vi "multiple_food.vi"(11 "pieceOfWorld in":T2[][](array[typedef])) -> (1 "columns":i32[](array[numeric]), 2 "rows":i32[](array[numeric]), 3 "foodAmount":T1)   [LabVIEW 2015, in "PolyVIEW.lvclass"]
uses:
  PolyVIEW.lvclass
  actors/world/typedefs/worldCell_cluster.ctl
  actors/world/typedefs/markValue_cluster.ctl
  actors/world/typedefs/markValue.ctl
  actors/world/typedefs/markVolume.ctl
  actors/world/typedefs/amountOfFood.ctl
  actors/world/typedefs/anthillType_enum.ctl
  actors/world/world.lvlib
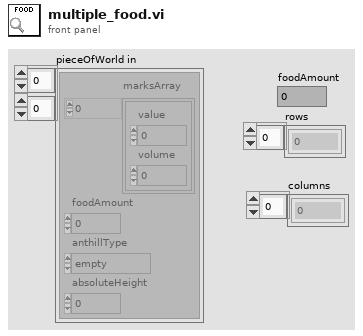
[diagram p1: front panel]
types:
  T1 = typedef "world.lvlib/amountOfFood.ctl" = i32
  T2 = typedef "world.lvlib/worldCell_cluster.ctl" = cluster{"marksArray":T3[], "foodAmount":T1, "anthillType":T6, "absoluteHeight":u8}
  T3 = typedef "world.lvlib/markValue_cluster.ctl" = cluster{"value":T4, "volume":T5}
  T4 = typedef "world.lvlib/markValue.ctl" = u8
  T5 = typedef "world.lvlib/markVolume.ctl" = u16
  T6 = typedef "world.lvlib/anthillType_enum.ctl" = enum16{"empty", "own", "rival"}
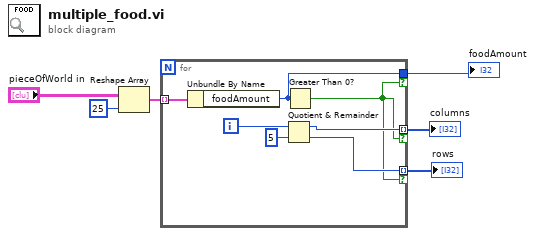
[diagram p0: block diagram]
diagram:
  n1 = Reshape Array("pieceOfWorld in", 25 ("dimension size")) -> (w5:T2[])
  n2 = for {
    tunnel: w5 -> [w13] mode=indexing
    tunnel: [w12] -> w3 if=w7
    tunnel: [w9] -> w2 mode=indexing if=w7
    tunnel: [w8] -> w1 mode=indexing if=w7
    i -> [w10]
    n3 = Unbundle By Name(w13) -> ("foodAmount"=w12:T1)
    n4 = Quotient & Remainder(x=w10, y=5) -> (x-y*floor(x/y)=w9:i32, floor(x/y)=w8:i32)
    n5 = Greater Than 0?(x=w12) -> (x > 0?=w7:bool)
  }
  "foodAmount" <- w3
  "columns" <- w2
  "rows" <- w1
